vi "VI_Heat_Tape_Final_subVI_final.vi"() -> ()   [LabVIEW 2019]
uses:
  <vilib>/NI/Modbus Library/API/Wrapper/Create Serial Master.vi
  <vilib>/NI/Modbus Library/API/Master/Modbus Master.lvclass
  <vilib>/NI/Modbus Library/API/Wrapper/API Main.lvlib
panel:
  in  "error check 2":errorcluster
  in  "COM Port (Station 02)":refnum<visa-resource-name>
  in  "Hysterisis (Station 02)":string
  in  "Set Value (Station 02)":string
  out "Connection (Station 02)":bool
  out "Current Temperature (ºF) 2":string
  out "Heat Tape 01  Temperature (ºF) 2":dbl(slide) scale=66.0..86.0
  in  "Hysterisis (Station 01)":string
  out "Connection Status (Station 01)":bool
  in  "Set Value (Station 01)":string
  in  "COM Port (Station 01)":refnum<visa-resource-name>
  out "?":cluster{dbl, dbl, dbl, dbl}(graph)
  in  "?":bool
  out "Current Temperature (ºF)":string
  out "Heat Tape Temperature Profiles (ºF)":dbl(slide) scale=65.0..85.0
  in  "error check":errorcluster
  # "SpinQuest Heat Tape Temperature Monitoring System"
  # "RS-485 Connections"
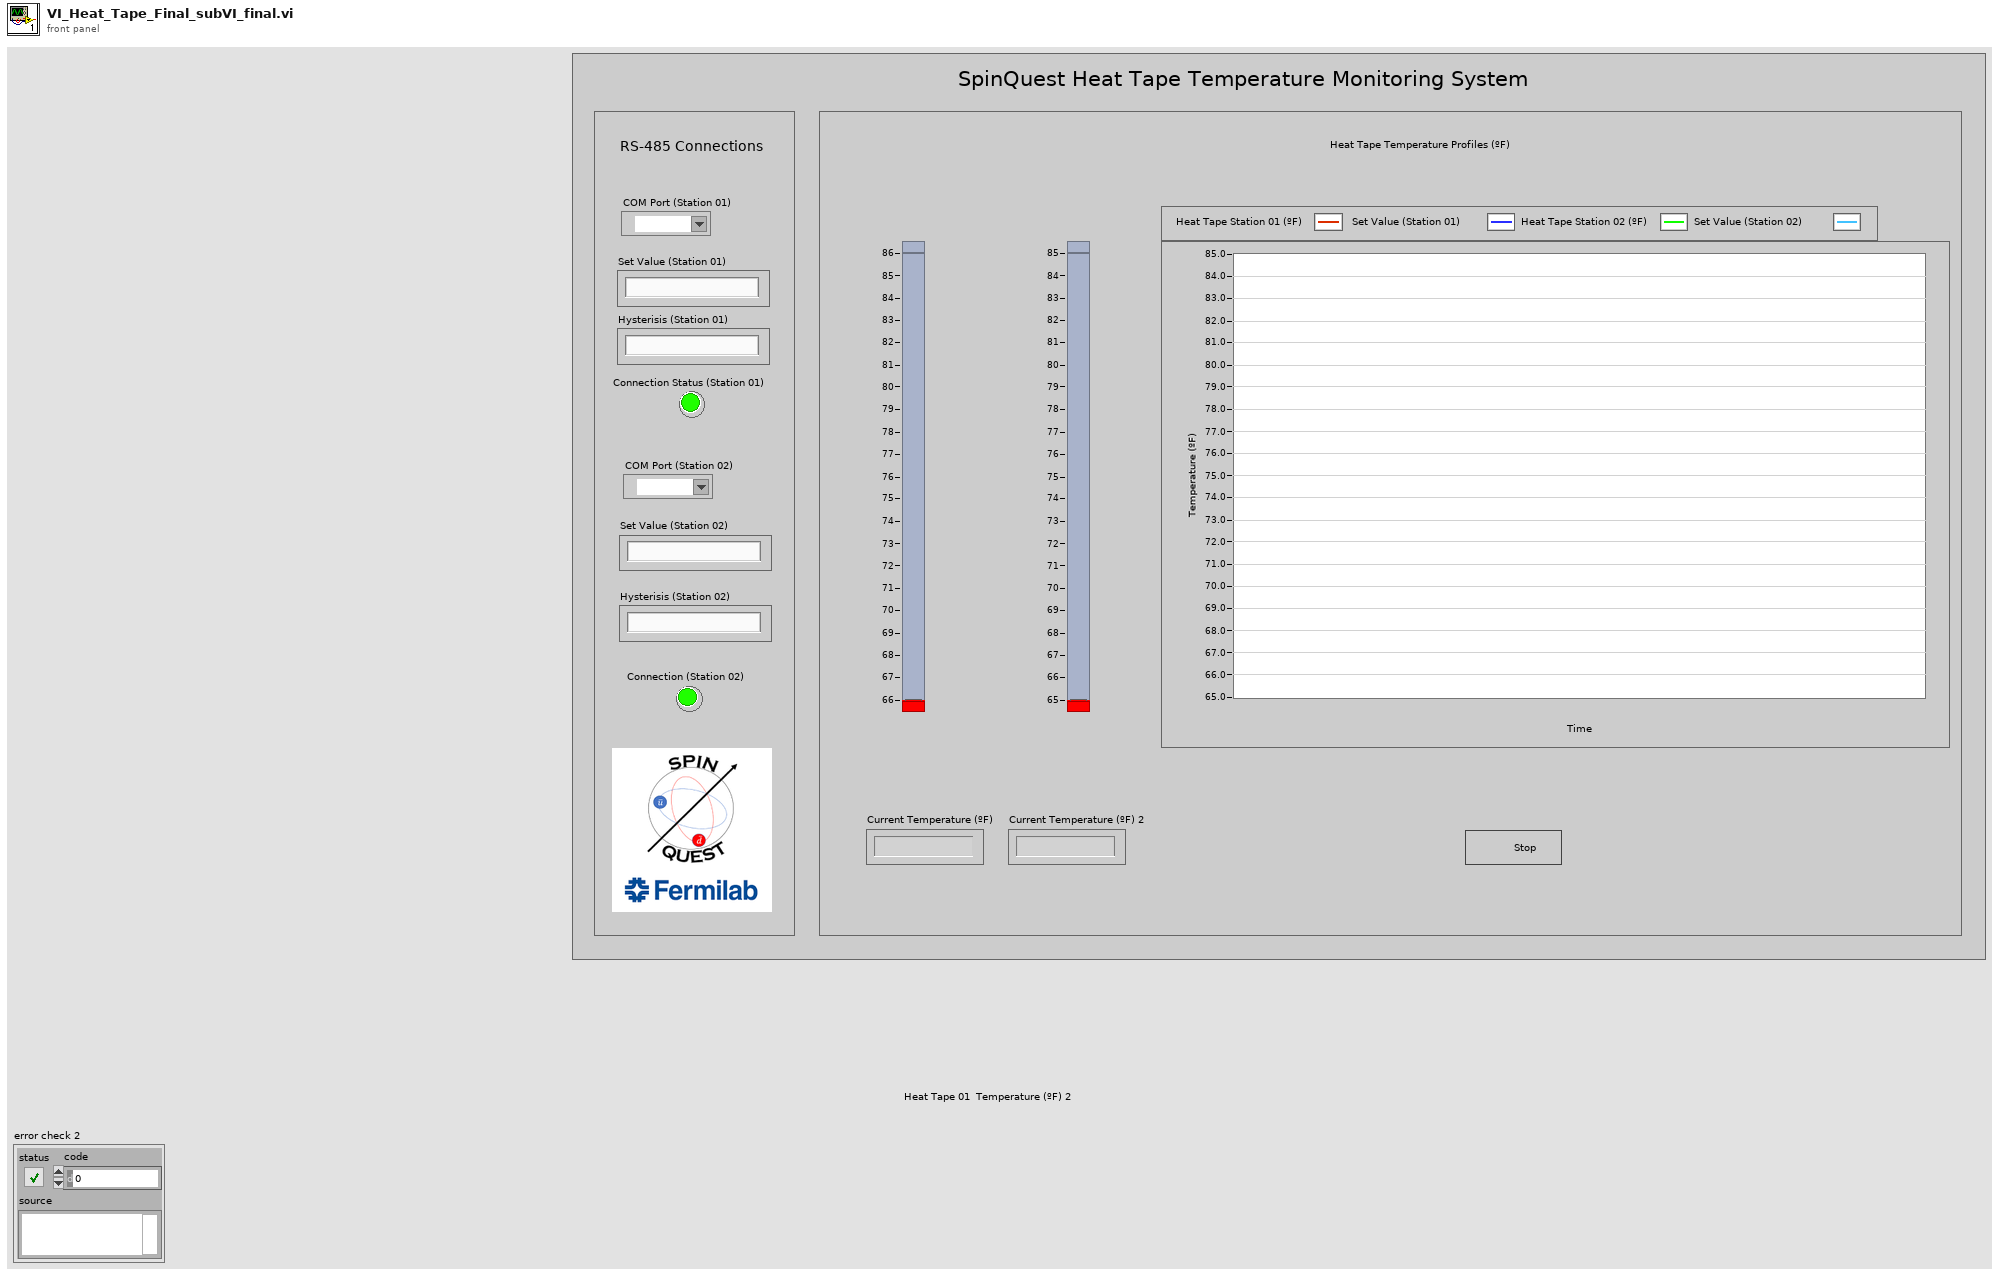
[diagram p1: front panel]
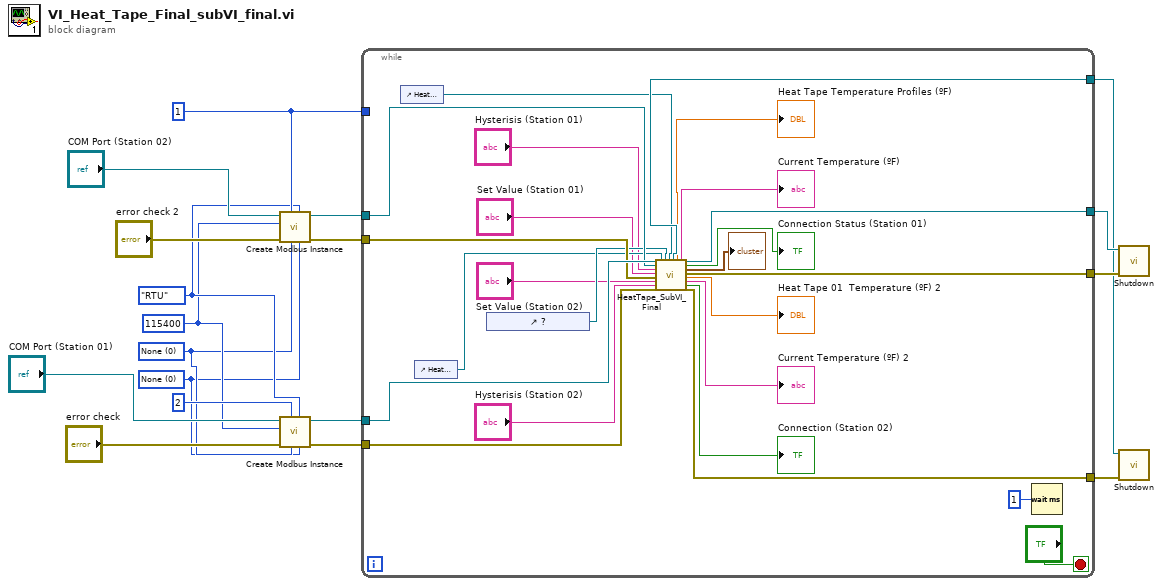
[diagram p0: block diagram]
diagram:
  w5 = u8 1 ("unit ID (Defaut: 1)")
  w4 = enum16{"RTU", "ASCII"}."RTU" ("Serial Type (Default: RTU)")
  w3 = u32 115400 ("Baud Rate (Default: 115400)")
  w1 = u16 0 items=["None", "XON/XOFF", "RTS/CTS", "XON/XOFF & RTS/CTS", "DTR/DSR", "XON/XOFF & DTR/DSR"] ("Flow Control (Default: None)")
  w2 = u16 0 items=["None", "Odd", "Even", "Mark", "Space"] ("Parity (Default: None)")
  n1 = call-poly <vilib>:"Create Modbus Instance.vi"("flow control (none)"=w1, "serial type"=w4, "parity (even)"=w2, "unit ID"=w5, "error in"="error check 2", "baud rate"=w3, "VISA resource name"="COM Port (Station 02)") -> ("error out"=w8:errorcluster, "serial master instance"=w7:refnum<class "Modbus Master.lvclass">)  [unwired: 3 in]
  n2 = call-poly <vilib>:"Create Modbus Instance.vi"("flow control (none)"=w1, "serial type"=w4, "parity (even)"=w2, "unit ID"=u8 2 ("unit ID (Defaut: 1)"), "error in"="error check", "baud rate"=w3, "VISA resource name"="COM Port (Station 01)") -> ("error out"=w16:errorcluster, "serial master instance"=w17:refnum<class "Modbus Master.lvclass">)  [unwired: 3 in]
  n3 = while {
    tunnel: w17 -> [w40]
    tunnel: w16 -> [w41]
    tunnel: [w39] -> w13
    tunnel: [w38] -> w12
    tunnel: [w37] -> w11
    tunnel: [w36] -> w10
    tunnel: w8 -> [w34]
    tunnel: w7 -> [w35]
    tunnel: w5 -> [_]
    stop <- "?" stop-if-true
    n4 = control-ref of="Heat Tape Temperature Profiles (ºF)"() -> (w33:refnum<vi>)
    n5 = control-ref of="Heat Tape 01  Temperature (ºF) 2"() -> (w31:refnum<vi>)
    n6 = control-ref of="?"() -> (w32:refnum<vi>)
    n7 = call "HeatTape_SubVI_Final.vi"("Modbus Master in"=w40, "serial master instance"=w35, "Hysterisis (Station 01)"="Hysterisis (Station 01)", "Set Value (Station 01)"="Set Value (Station 01)", "error in"=w34, "Set Value (Station 02)"="Set Value (Station 02)", "Hysterisis (Station 02)"="Hysterisis (Station 02)", "error in (no error)"=w41, "Slide Refnum 2"=w31, "WFChart Refnum"=w32, "Slide Refnum"=w33) -> ("Modbus master out"=w37:refnum<class "Modbus Master.lvclass">, "Numeric"=→"Heat Tape Temperature Profiles (ºF)":dbl, "String 2"=→"Current Temperature (ºF)":string, "Modbus Master out"=w39:refnum<class "Modbus Master.lvclass">, "Boolean"=→"Connection Status (Station 01)":bool, "Cluster"=→"?":cluster{dbl, dbl, dbl, dbl}, "error out 3"=w38:errorcluster, "Numeric 2"=→"Heat Tape 01  Temperature (ºF) 2":dbl, "String"=→"Current Temperature (ºF) 2":string, "Boolean 2"=→"Connection (Station 02)":bool, "error out"=w36:errorcluster)  [unwired: 6 in]
    n8 = Wait (ms)(milliseconds to wait=u32 1) -> ()  [unwired: 1 out]
  }
  n9 = call-dynamic "Shutdown.vi"("error in"=w12, "Modbus master in"=w13) -> ()  [unwired: 9 in, 1 out]
  n10 = call-dynamic "Shutdown.vi"("error in"=w10, "Modbus master in"=w11) -> ()  [unwired: 9 in, 1 out]
